vi "S&E Event String.vi"(2 "Elevated priority":bool, 7 "Content":variant, 9 "error in":errorcluster) -> (8 "format string":string, 10 "error out":errorcluster)   [LabVIEW 2011]
uses:
  reate/S&E Event Type.ctl
  reate/S&E Event source.ctl
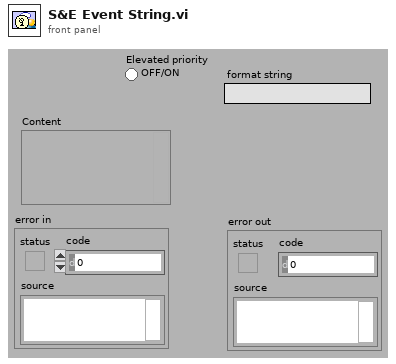
[diagram p1: front panel]
types:
  T1 = typedef "S&E Event Type.ctl" = cluster{"Event Source":T2, "Source Info":string, "Event Description":string}
  T2 = typedef "S&E Event source.ctl" = enum16{"User", "Instrument", "Application", "Windows"}
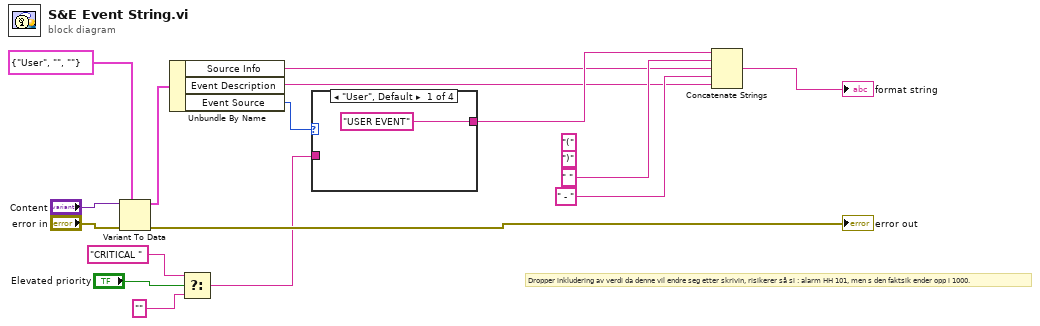
[diagram p0: block diagram]
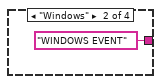
[diagram p2: hidden frame]
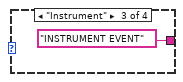
[diagram p3: hidden frame]
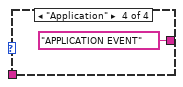
[diagram p4: hidden frame]
diagram:
  (unwired) ")" ("string")
  (unwired) "(" ("string")
  # "Dropper inkludering av verdi da denne vil endre seg etter skrivin, risikerer så si : alarm HH 101, men s den faktsik ender opp i 1000."
  n1 = Variant To Data(error in="error in", type=T1 {"Event Source"=enum."User", "Source Info"="", "Event Description"=""} ("S&E Event"), Variant="Content") -> (data=w12:T1, error out=→"error out":errorcluster)
  n2 = Unbundle By Name(w12) -> ("Source Info"=w2:string, "Event Description"=w1:string, "Event Source"=w8:T2)
  n3 = Select(t="CRITICAL " ("string"), s="Elevated priority", f="") -> (s? t:f=w4:string)
  n4 = case shown="\"User\", Default" w8 {
    tunnel: ["USER EVENT" ("string") "WINDOWS EVENT" ("string") "INSTRUMENT EVENT" ("string") "APPLICATION EVENT" ("string")] -> w3
    tunnel: w4 -> [_ _ _ _]
    frame "User", Default {
    }
    frame "Windows" {
    }
    frame "Instrument" {
    }
    frame "Application" {
    }
  }
  n5 = Concatenate Strings(w3, " " ("string"), w2, " - " ("string"), w1) -> (→"format string":string)
